vi "Periodic Tasks.vi"(8 "error in":errorcluster) -> ()   [LabVIEW 2012]
doc: "This VI runs in parallel to other tasks. It can contain as many user-defined periodic loops as you need. These can carry out PID or other sorts of timed response."
uses:
  <vilib>/Rock Robotics/SystemInterfaces/Utilities/FPGA_UtilitiesLED Source.ctl
  <vilib>/Rock Robotics/SystemInterfaces/Utilities/FPGA_UtilitiesLED State.ctl
  <vilib>/Rock Robotics/WPI/Compressor/WPI_CompressorGetSetRefNum.vi
  Robot Global Data.vi
panel:
  out "Compressor Loop Running":bool
  out "Compressor Running":bool
  out "Compressor Enabled":bool
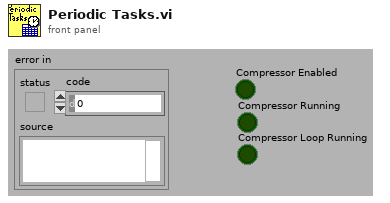
[diagram p1: front panel]
types:
  T1 = typedef "FPGA_UtilitiesLED State.ctl" = enum16{"Off", "On", "Toggle"}
  T2 = typedef "FPGA_UtilitiesLED Source.ctl" = enum16{"User LED", "FPGA LED"}
  T3 = typedef "WPI_CompressorDevRef.ctl" = cluster{"DevStatus":errorcluster, "DigitalInputDevRef":T4, "RelayDevRef":T7}
  T4 = typedef "WPI_DigitalInputDevRef.ctl" = cluster{"DevStatus":errorcluster, "DIO Channel":T5, "Digital Module":T6}
  T5 = typedef "FPGA_DIOChannel.ctl" = enum8{"DIO 1", "DIO 2", "DIO 3", "DIO 4", "DIO 5", "DIO 6", "DIO 7", "DIO 8", "DIO 9", "DIO 10", "DIO 11", "DIO 12", "DIO 13", "DIO 14", "Invalid"}
  T6 = typedef "FPGA_TypedefDigitalModule.ctl" = enum16{"Digital Module 1", "Digital Module 2"}
  T7 = typedef "WPI_RelayDevRef.ctl" = cluster{"DevStatus":errorcluster, "Relay Channel":T8, "Digital Module":T6, "Relay Direction":T9}
  T8 = typedef "FPGA_DIORelayChannel.ctl" = enum8{"Relay 1", "Relay 2", "Relay 3", "Relay 4", "Relay 5", "Relay 6", "Relay 7", "Relay 8", "Invalid"}
  T9 = typedef "WPI_RelayDirection.ctl" = enum16{"Both directions", "Forward only", "Reverse only"}
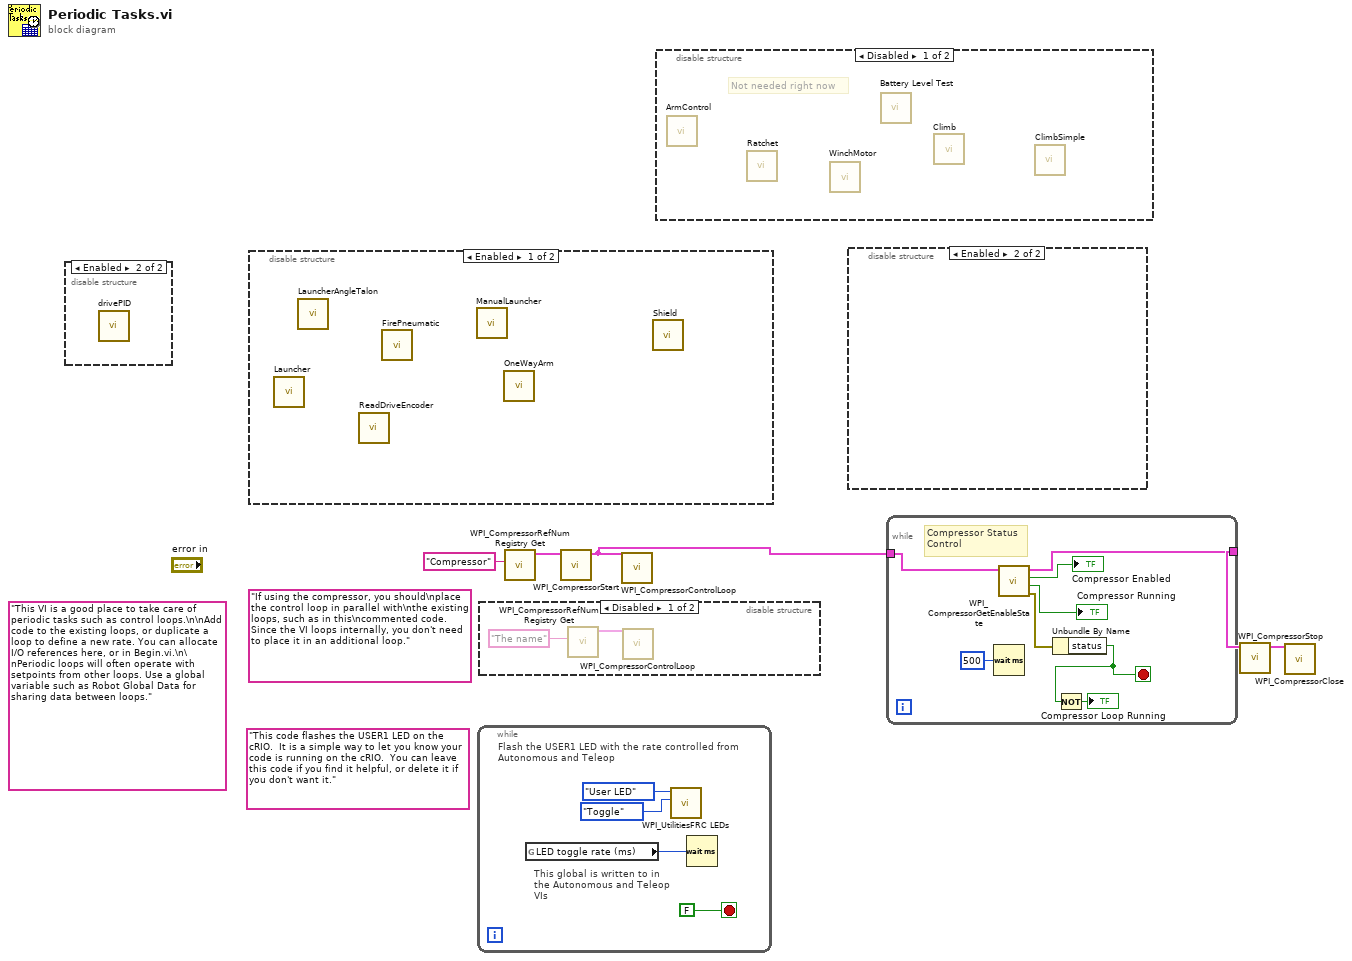
[diagram p0: block diagram]
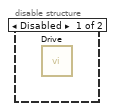
[diagram p2: hidden frame]
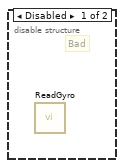
[diagram p4: hidden frame]
diagram:
  (unwired) "If using the compressor, you should\nplace the control loop in parallel with\nthe existing loops, such as in this\ncommented code. Since the VI loops internally, you don't need to place it in an additional loop."
  (unwired) "This code flashes the USER1 LED on the cRIO.  It is a simple way to let you know your code is running on the cRIO.  You can leave this code if you find it helpful, or delete it if you don't want it."
  (unwired) "This VI is a good place to take care of periodic tasks such as control loops.\n\nAdd code to the existing loops, or duplicate a loop to define a new rate. You can allocate I/O references here, or in Begin.vi.\n\nPeriodic loops will often operate with setpoints from other loops. Use a global variable such as Robot Global Data for sharing data between loops."
  n1 = disable-structure shown="Enabled" {
    frame Disabled {
      n2 = call "Drive.vi"() -> ()  [unwired: 12 in]
    }
    frame Enabled {
      n3 = call "drivePID.vi"() -> ()  [unwired: 12 in]
    }
  }
  n4 = disable-structure shown="Enabled" {
    frame Enabled {
      n5 = call "Launcher.vi"() -> ()  [unwired: 12 in]
      n6 = call "LauncherAngleTalon.vi"() -> ()  [unwired: 12 in]
      n7 = call "ReadDriveEncoder.vi"() -> ()  [unwired: 12 in]
      n8 = call "FirePneumatic.vi"() -> ()  [unwired: 12 in]
      n9 = call "ManualLauncher.vi"() -> ()  [unwired: 12 in]
      n10 = call "OneWayArm.vi"() -> ()  [unwired: 12 in]
      n11 = call "Shield.vi"() -> ()  [unwired: 12 in]
    }
    frame Disabled {
    }
  }
  n12 = while {
    stop <- FALSE stop-if-true
    # "This global is written to in the Autonomous and Teleop VIs"
    # "Flash the USER1 LED with the rate controlled from Autonomous and Teleop"
    n13 = global read "Robot Global Data.vi" "LED toggle rate (ms)"() -> (w6:u32)
    n14 = call <vilib>:"WPI_UtilitiesFRC LEDs.vi"("State"=FPGA_UtilitiesLED_State."Toggle", "LED Type"=FPGA_UtilitiesLED_Source."User LED") -> ()  [unwired: 1 in, 9 out]
    n15 = Wait (ms)(milliseconds to wait=w6) -> ()  [unwired: 1 out]
  }
  n16 = disable-structure shown="Disabled" {
    frame Disabled {
      n17 = call <vilib>:"WPI_CompressorRefNum Registry Get.vi"("refnum name"="The name") -> ("CompressorDevRef"=w11:T3)  [unwired: 9 in, 1 out]
      n18 = call <vilib>:"WPI_CompressorControlLoop.vi"("CompressorDevRef"=w11) -> ()  [unwired: 11 in]
    }
    frame Enabled {
    }
  }
  n19 = call <vilib>:"WPI_CompressorRefNum Registry Get.vi"("refnum name"="Compressor") -> ("CompressorDevRef"=w5:T3)  [unwired: 9 in, 1 out]
  n20 = call <vilib>:"WPI_CompressorStart.vi"("CompressorDevRef"=w5) -> ("CompressorDevRef"=w3:T3)  [unwired: 9 in, 1 out]
  n21 = call <vilib>:"WPI_CompressorControlLoop.vi"("CompressorDevRef"=w3) -> ()  [unwired: 11 in]
  n22 = disable-structure shown="Disabled" {
    frame Disabled {
      # "Not needed right now"
      n23 = call "ArmControl.vi"() -> ()  [unwired: 12 in]
      n24 = call "Ratchet.vi"() -> ()  [unwired: 12 in]
      n25 = call "WinchMotor.vi"() -> ()  [unwired: 12 in]
      n26 = call "Battery Level Test.vi"() -> ()  [unwired: 12 in]
      n27 = call "Climb.vi"() -> ()  [unwired: 12 in]
      n28 = call "ClimbSimple.vi"() -> ()  [unwired: 12 in]
    }
    frame Enabled {
    }
  }
  n29 = disable-structure shown="Enabled" {
    frame Disabled {
      # "Bad"
      n30 = call "ReadGyro.vi"() -> ()  [unwired: 12 in]
    }
    frame Enabled {
    }
  }
  n31 = while {
    tunnel: w3 -> [w19]
    tunnel: [w14] -> w2
    stop <- w12 stop-if-true
    # "Compressor Status\nControl"
    n32 = Wait (ms)(milliseconds to wait=u32 500) -> ()  [unwired: 1 out]
    n33 = call <vilib>:"WPI_CompressorGetEnableState.vi"("CompressorDevRef"=w19) -> ("error out"=w15:errorcluster, "Compressor Running"=→"Compressor Running":bool, "Enabled"=→"Compressor Enabled":bool, "CompressorDevRef"=w14:T3)  [unwired: 1 in, 6 out]
    n34 = Unbundle By Name(w15) -> ("status"=w12:bool)
    n35 = Not(x=w12) -> (.not. x?=→"Compressor Loop Running":bool)
  }
  n36 = call <vilib>:"WPI_CompressorStop.vi"("CompressorDevRef"=w2) -> ("CompressorDevRef"=w1:T3)  [unwired: 1 in, 9 out]
  n37 = call <vilib>:"WPI_CompressorClose.vi"("CompressorDevRef"=w1) -> ()  [unwired: 1 in, 10 out]
